vi "UI-抓边计算壁厚.vi"(8 "error in (no error)":errorcluster caption="错误输入（无错误）", 11 "名称或相对路径":string="Template Program") -> (0 "error in (no error) 2":errorcluster caption="错误输入（无错误）")   [LabVIEW 2017]
uses:
  Global System.vi
  <vilib>/Utility/xml.llb/Read From XML File(string).vi
  <vilib>/Utility/xml.llb/Write to XML File(string).vi
  Picture/SaveButtom.ctl
  <vilib>/vision/Measure.llb/Edge Polarity.ctl
  <vilib>/vision/Measure.llb/Edge Options.ctl
panel:
  out "添加的路径":path
  in  "刷新":bool
  in  "测试按钮":bool
  in  "保存按钮":bool
  in  "Main":enum32{"主参数", "计算圆心参数 ", "边界检查器设定", "测试效果"}(tab)
  in  "ParamsUI":T1={"IsNorImage"=TRUE, "Exposure Values"=100289, "ImagePath"=path "C:/Users/hedongpo/Desktop/514-hdp/Alignment Assemble System/Test Picture/B/3.bmp"} caption="参数界面" {"Exposure Values" scale=0.0..200000.0}
  in  "ParamsUI 内圆":T5={"圆参数1"={"Search  Direction"=0, "Edge Options"={"Edge Polarity"=0, "Kernel Size"=3, "Width"=3, "Minimum Edge Strength"=50.0, "Interpolation Type"=enum."Bilinear Fixed", "Data Processing Method"=enum."Average"}, "Show Search Area"=TRUE, "Show Search Lines"=TRUE, "Show Edges Found"=TRUE, "Show Result"=TRUE, "Search Area Color"=65280, "Search Lines Color"=255, "Edge Locations Color"=16776960, "Result Color"=16711680, "Overlay Group Name"=""}, "圆参数"={"Process"=enum."Get First Edge", "Step Size"=1, "Max Pixel Radius"=3}, "圆二值化设定"={"Lower value"=96.0, "Upper value"=255.0}, "圆环ROI设定"={"Center X"=1717, "Center Y"=1486, "Inner Radius"=327, "Outer Radius"=1645, "Start Angle"=0.0, "End Angle"=0.0}, "Show Search Area"=TRUE, "Show Search Lines"=TRUE, "Show Edges Found"=TRUE, "Show Result"=TRUE} caption="参数界面" {"圆环ROI设定"."End Angle" min=-90.0 max=90.0 step=1.0 format="%.2f"; "圆环ROI设定"."Start Angle" min=-90.0 max=90.0 step=1.0 format="%.2f"; "圆环ROI设定"."Center X" scale=0.0..1024.0; "圆参数1"."Search  Direction" items=["Outside to Inside", "Inside to Outside"]; "圆参数1"."Edge Options"."Edge Polarity" items=["All Edges", "Rising Edges", "Falling Edges"]; "圆参数1"."Edge Options"."Minimum Edge Strength" format="%.2f"; "圆参数1"."Edge Options"."Width" step=2; "圆参数1"."Edge Options"."Kernel Size" step=2}
  in  "ParamsUI 边界检查器":T6={"外圆二值化设定"={"Lower value"=96.0, "Upper value"=255.0}, "扇区个数"="1", "Process "=enum."Get All Edges", "Edge Options "={"Edge Polarity"=0, "Kernel Size"=9, "Width"=5, "Minimum Edge Strength"=27.0, "Interpolation Type"=enum."Bilinear", "Data Processing Method"=enum."Average"}} caption="参数界面" {"Edge Options"."Edge Polarity" items=["All Edges", "Rising Edges", "Falling Edges"]}
  out "壁厚波形图":sgl[](graph)
  in  "测试结果":string[][](table)=[["", ""]]
  out "原始图像":T7(plugin-control)
  out "处理后图像":T7(plugin-control)
  out "路径输出":path
  in  "Vision Paramter Save Buttom":T8
  out "system time":string
  in  "取消按钮":bool
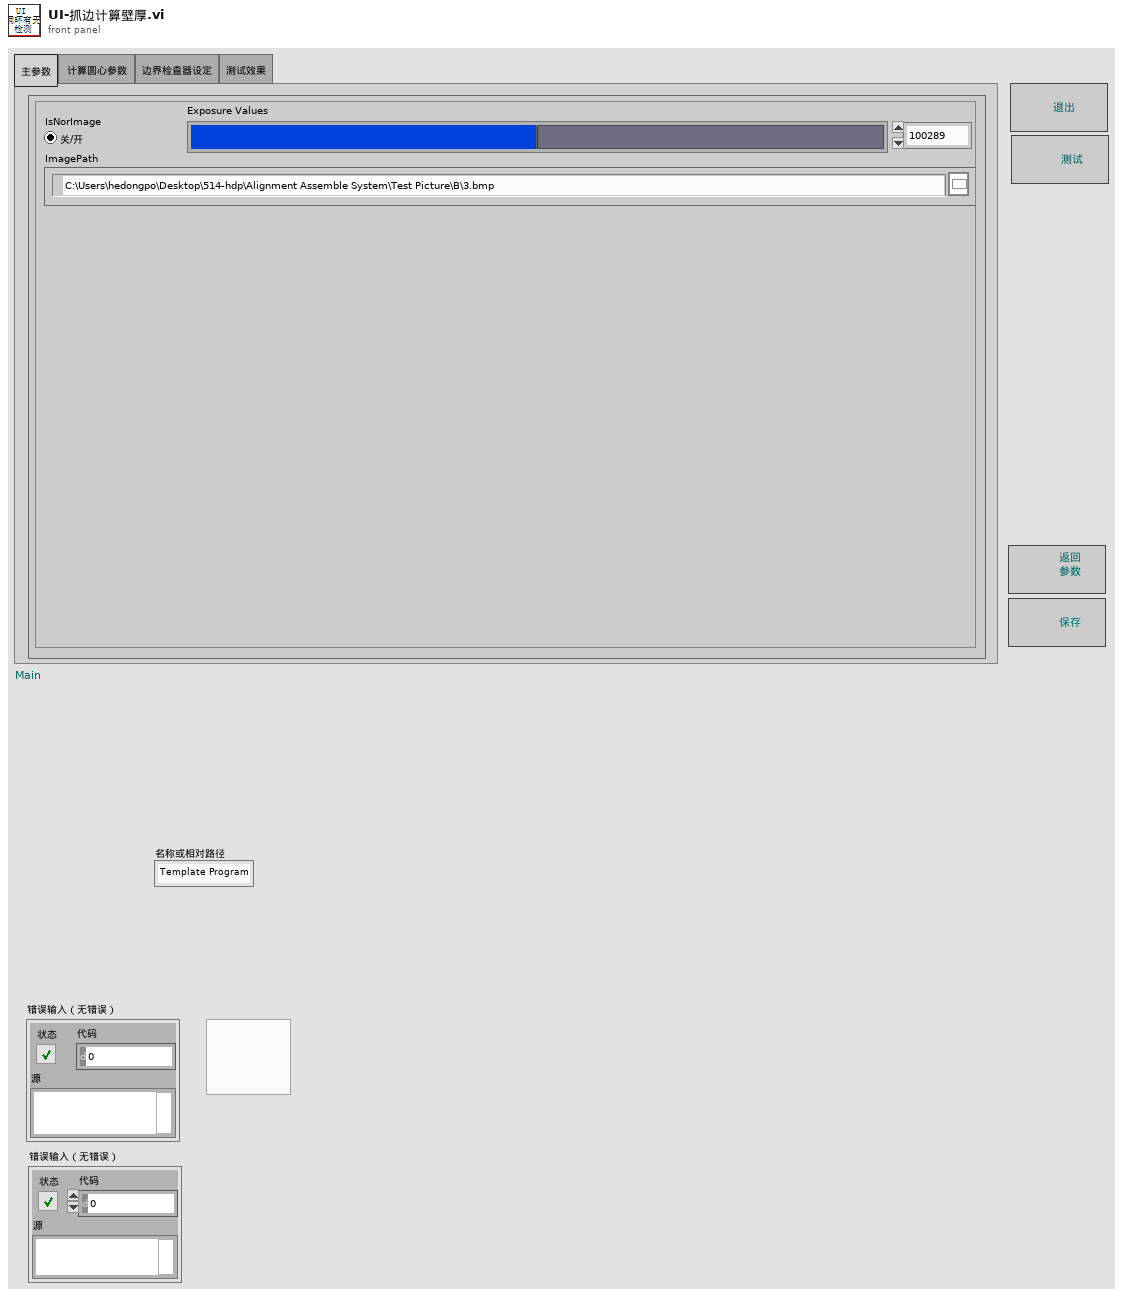
[diagram p1: front panel]
types:
  T1 = cluster{"IsNorImage":bool, "Exposure Values":u32, "ImagePath":path}
  T2 = typedef "Edge Options.ctl" = cluster{"Edge Polarity":T3, "Kernel Size":u32, "Width":u32, "Minimum Edge Strength":sgl, "Interpolation Type":enum32{"Zero Order", "Bilinear", "Quadratic", "Cubic", "Bilinear Fixed"}, "Data Processing Method":enum32{"Average", "Median"}}
  T3 = typedef "Edge Polarity.ctl" = u32
  T4 = typedef "IMAQ Circle" = cluster{"Center X":i32, "Center Y":i32, "Inner Radius":i32, "Outer Radius":i32, "Start Angle":dbl, "End Angle":dbl}
  T5 = cluster{"圆参数1":cluster{"Search  Direction":u32, "Edge Options":T2, "Show Search Area":bool, "Show Search Lines":bool, "Show Edges Found":bool, "Show Result":bool, "Search Area Color":u32, "Search Lines Color":u32, "Edge Locations Color":u32, "Result Color":u32, "Overlay Group Name":string}, "圆参数":cluster{"Process":enum16{"Get First Edge", "Get First + Last Edge", "Get All Edges", "Get Best Edge"}, "Step Size":i32, "Max Pixel Radius":i32}, "圆二值化设定":cluster{"Lower value":sgl, "Upper value":sgl}, "圆环ROI设定":T4, "Show Search Area":bool, "Show Search Lines":bool, "Show Edges Found":bool, "Show Result":bool}
  T6 = cluster{"外圆二值化设定":cluster{"Lower value":sgl, "Upper value":sgl}, "扇区个数":string, "Process ":enum16{"Get First Edge", "Get First + Last Edge", "Get All Edges", "Get Best Edge"}, "Edge Options ":cluster{"Edge Polarity":u32, "Kernel Size":u32, "Width":u32, "Minimum Edge Strength":sgl, "Interpolation Type":enum32{"Zero Order", "Bilinear", "Quadratic", "Cubic", "Bilinear Fixed"}, "Data Processing Method":enum32{"Average", "Median"}}}
  T7 = typedef "IMAQ Image.ctl" = refnum<image>
  T8 = typedef "SaveButtom.ctl" = bool
  T9 = cluster{"index":i32, "this vi":refnum<vi>, "error out":errorcluster}
  T10 = cluster{"master data":string, "priority":u16, "secondary data":string[]}
  T11 = cluster{"case name":string[], "queue array":refnum<queue>[]}
  T12 = cluster{"扇区个数":string, "Fitted Circle (Find Circular Edge 1)":cluster{"Center (Pixels)":cluster{"X":sgl, "Y":sgl}, "Radius (Pixels)":dbl, "Center (Real-World)":cluster{"X":sgl, "Y":sgl}, "Radius (Real-World)":dbl, "Roundness (Real-World)":dbl, "Average Strength":dbl, "Average SNR (dB)":dbl}, "Range (Threshold 1)":cluster{"Lower value":sgl, "Upper value":sgl}, "Process (Edge Detector 1)":enum16{"Get First Edge", "Get First + Last Edge", "Get All Edges", "Get Best Edge"}, "Edge Options (Edge Detector 1)":cluster{"Edge Polarity":u32, "Kernel Size":u32, "Width":u32, "Minimum Edge Strength":sgl, "Interpolation Type":enum32{"Zero Order", "Bilinear", "Quadratic", "Cubic", "Bilinear Fixed"}, "Data Processing Method":enum32{"Average", "Median"}}}
  T13 = typedef "Image Type" = u32
  T14 = cluster{"Search  Direction":u32, "Edge Options":T2, "Show Search Area":bool, "Show Search Lines":bool, "Show Edges Found":bool, "Show Result":bool, "Search Area Color":u32, "Search Lines Color":u32, "Edge Locations Color":u32, "Result Color":u32, "Overlay Group Name":string}
  T15 = cluster{"Process":enum16{"Get First Edge", "Get First + Last Edge", "Get All Edges", "Get Best Edge"}, "Step Size":i32, "Max Pixel Radius":i32}
  T16 = enum16{"Get First Edge", "Get First + Last Edge", "Get All Edges", "Get Best Edge"}
  T17 = cluster{"Edge Polarity":u32, "Kernel Size":u32, "Width":u32, "Minimum Edge Strength":sgl, "Interpolation Type":enum32{"Zero Order", "Bilinear", "Quadratic", "Cubic", "Bilinear Fixed"}, "Data Processing Method":enum32{"Average", "Median"}}
  T18 = typedef "ROI Descriptor" = cluster{"Global Rectangle":i32[], "Contours":cluster{"ID":enum32{"External", "Internal"}, "Type":u32, "Coordinates":i32[]}[]}
  T19 = cluster{"Center (Pixels)":cluster{"X":sgl, "Y":sgl}, "Radius (Pixels)":dbl, "Center (Real-World)":cluster{"X":sgl, "Y":sgl}, "Radius (Real-World)":dbl, "Roundness (Real-World)":dbl, "Average Strength":dbl, "Average SNR (dB)":dbl}
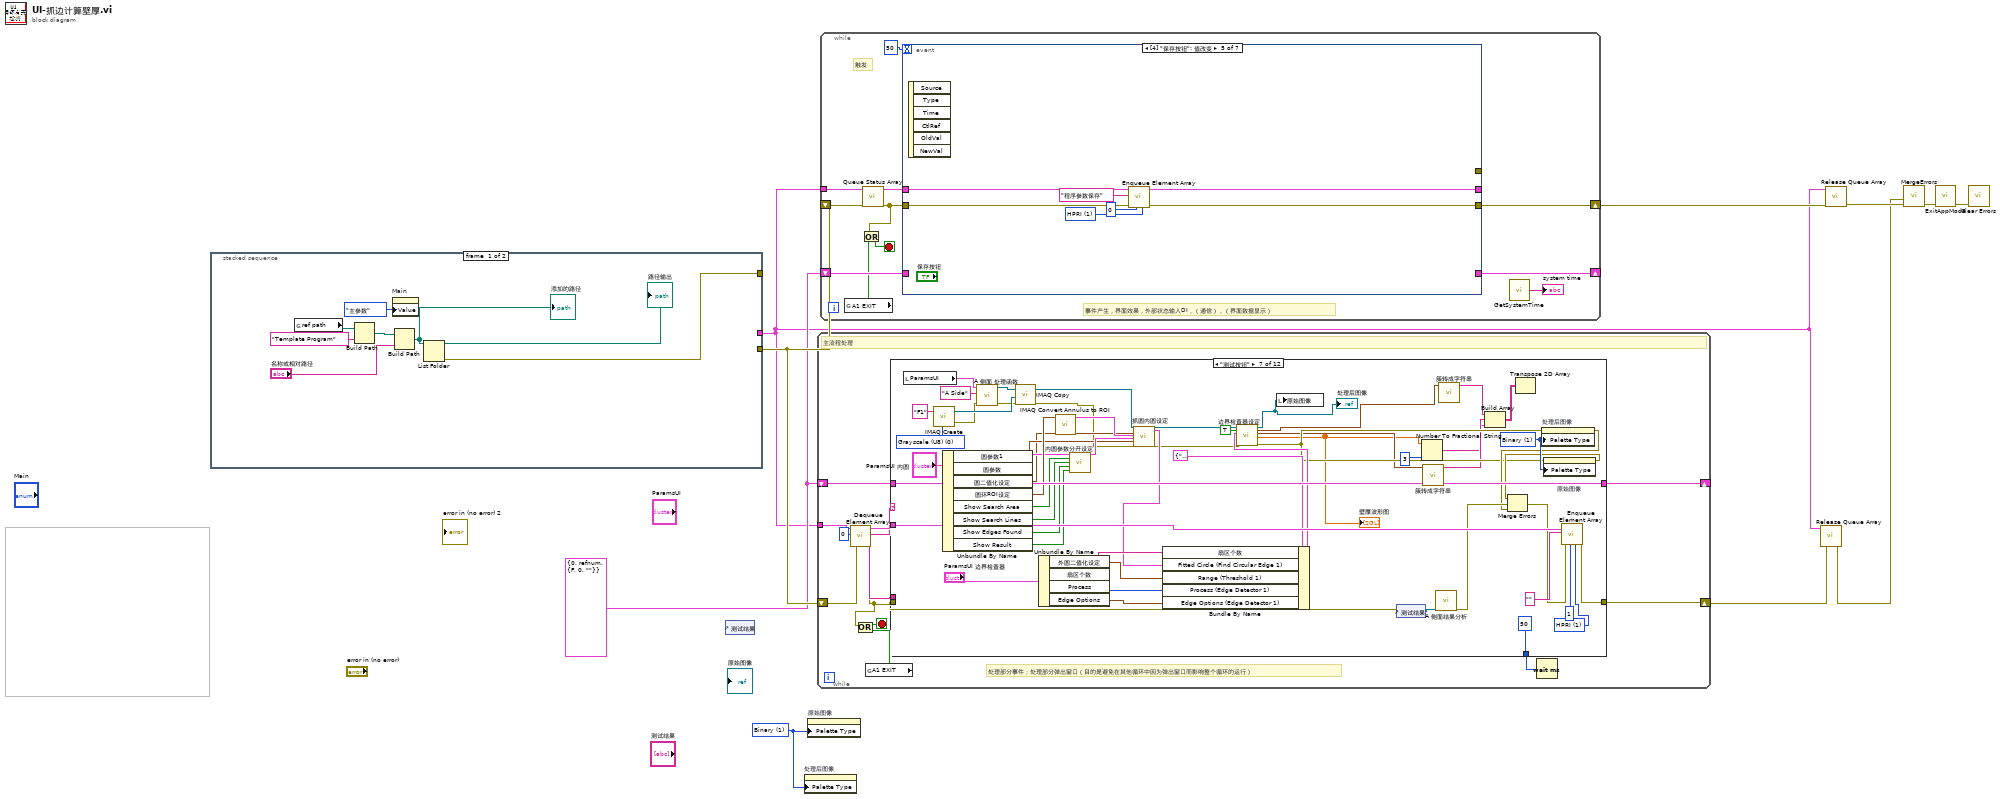
[diagram p0: block diagram]
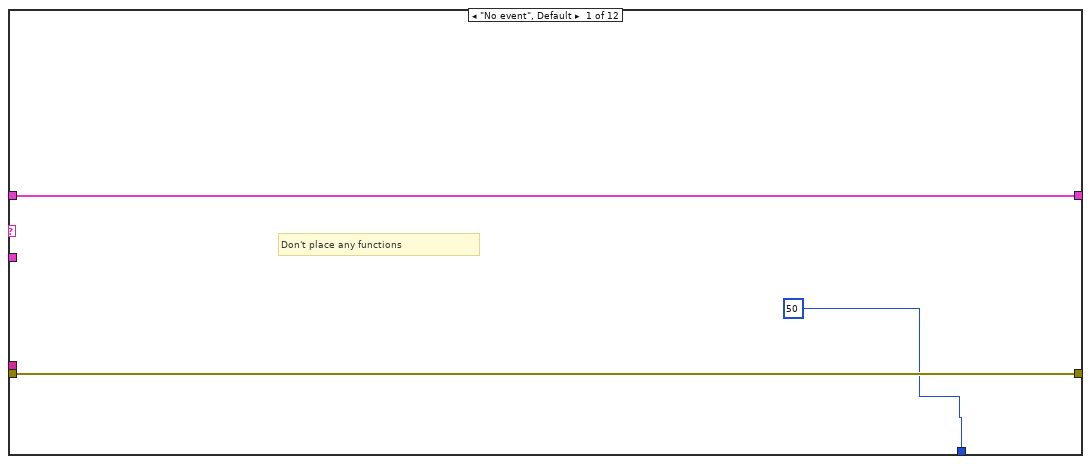
[diagram p2: hidden frame]
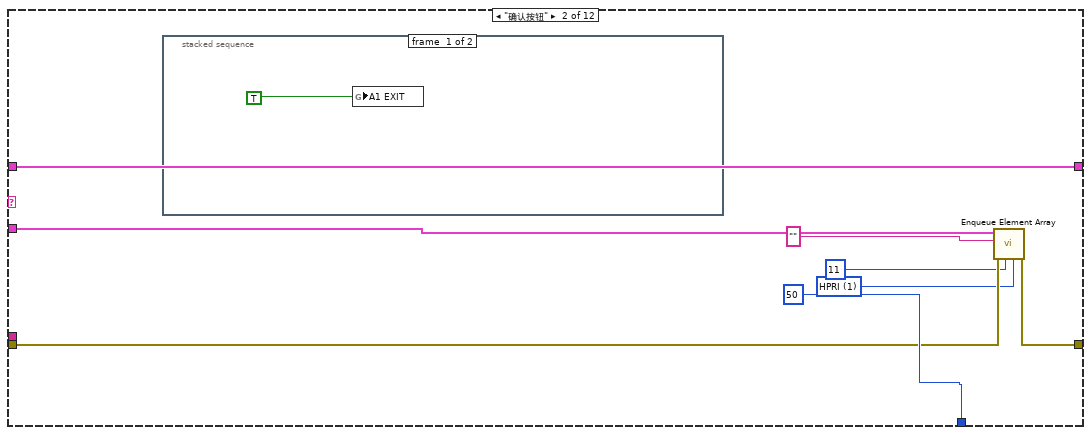
[diagram p3: hidden frame]
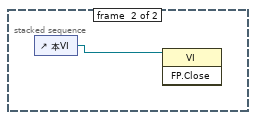
[diagram p4: hidden frame]
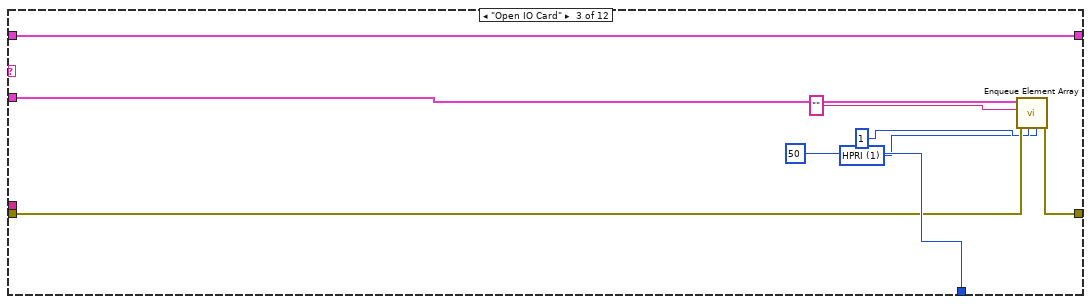
[diagram p5: hidden frame]
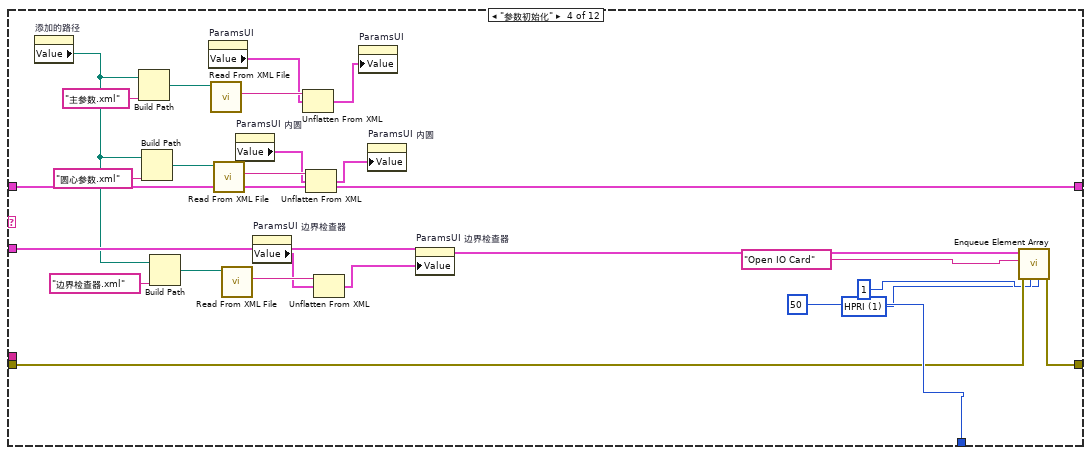
[diagram p6: hidden frame]
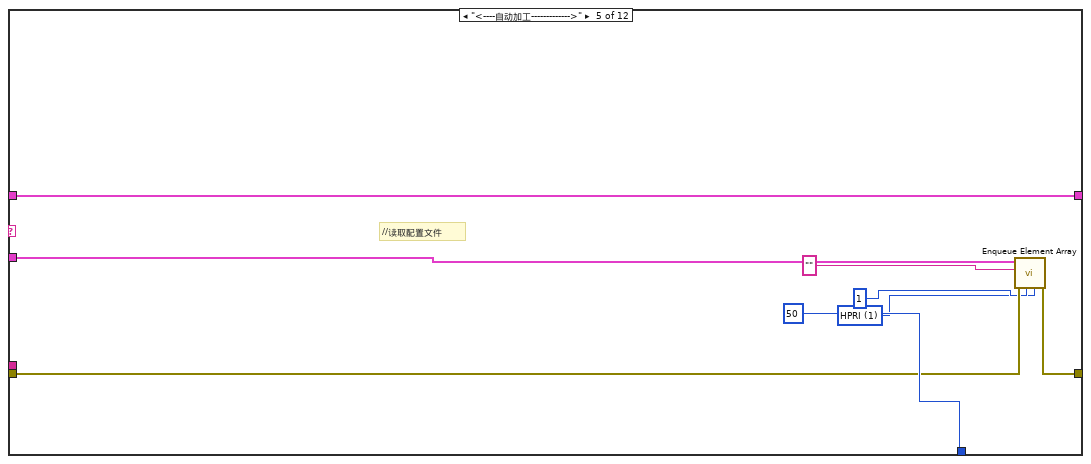
[diagram p7: hidden frame]
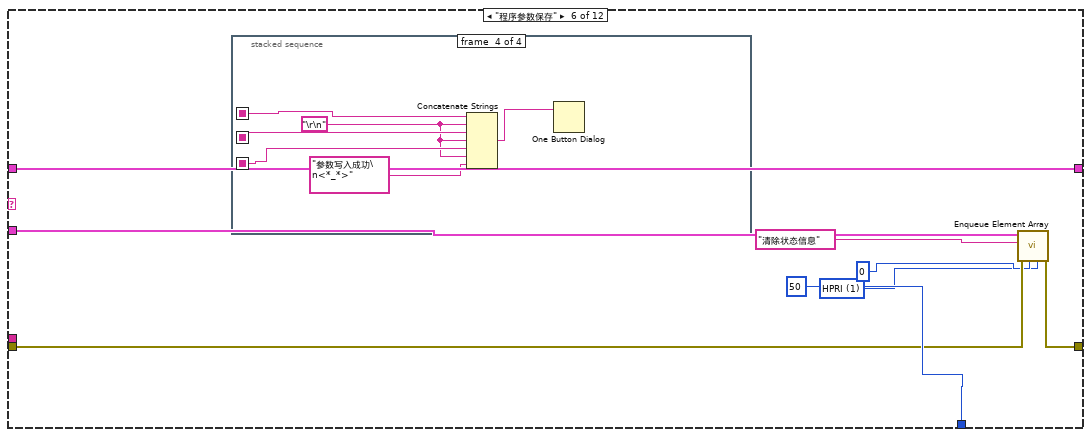
[diagram p8: hidden frame]
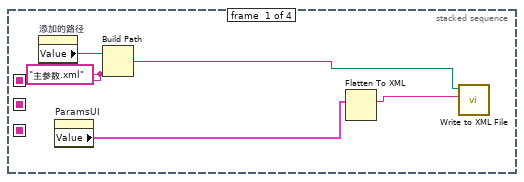
[diagram p9: hidden frame]
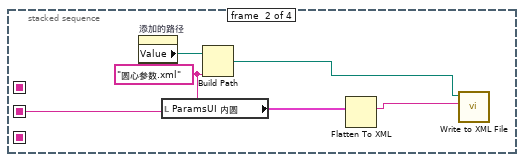
[diagram p10: hidden frame]
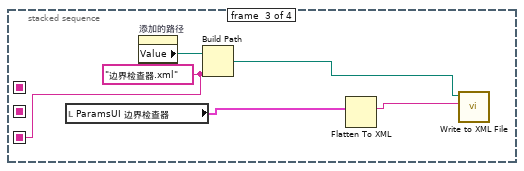
[diagram p11: hidden frame]
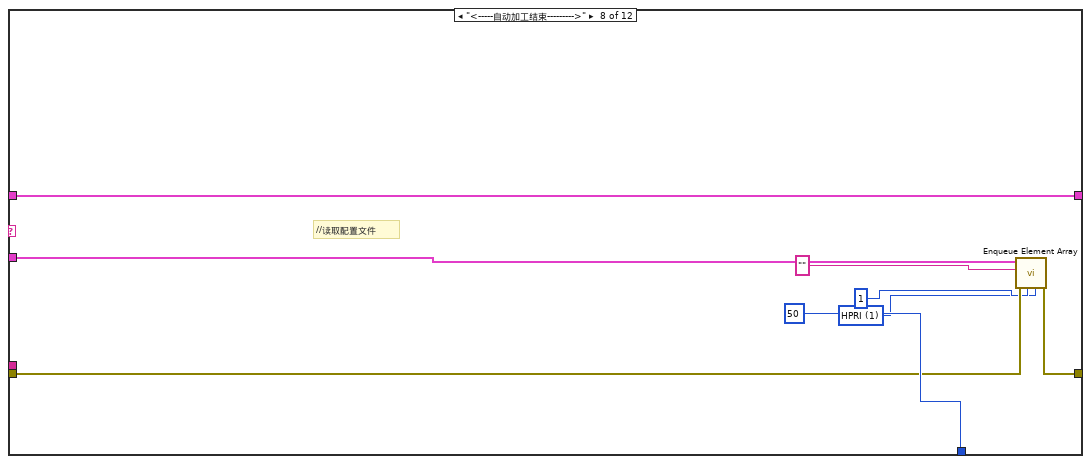
[diagram p12: hidden frame]
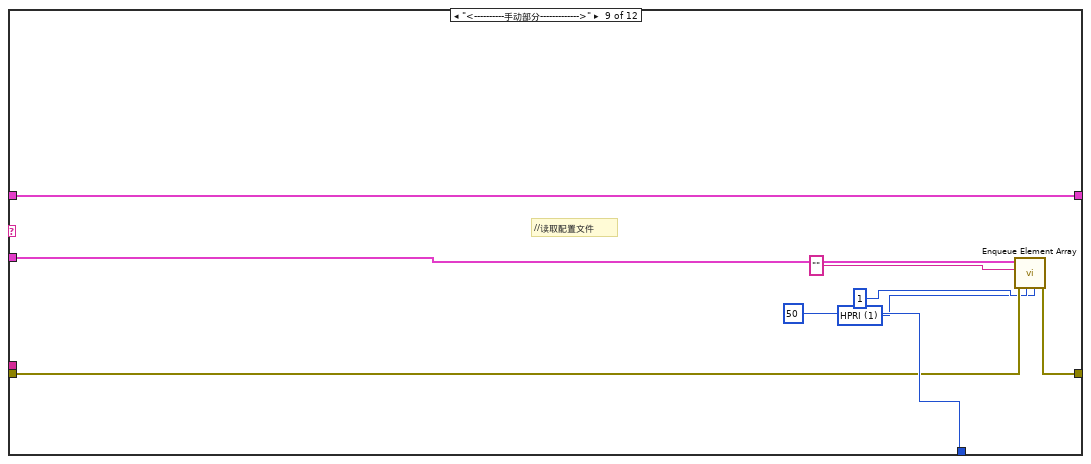
[diagram p13: hidden frame]
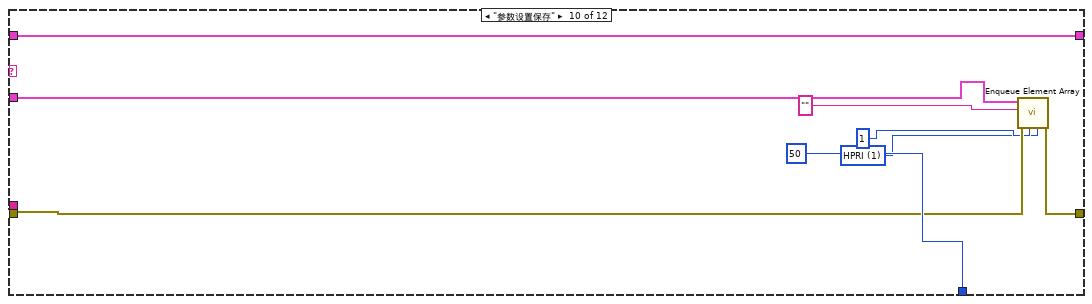
[diagram p14: hidden frame]
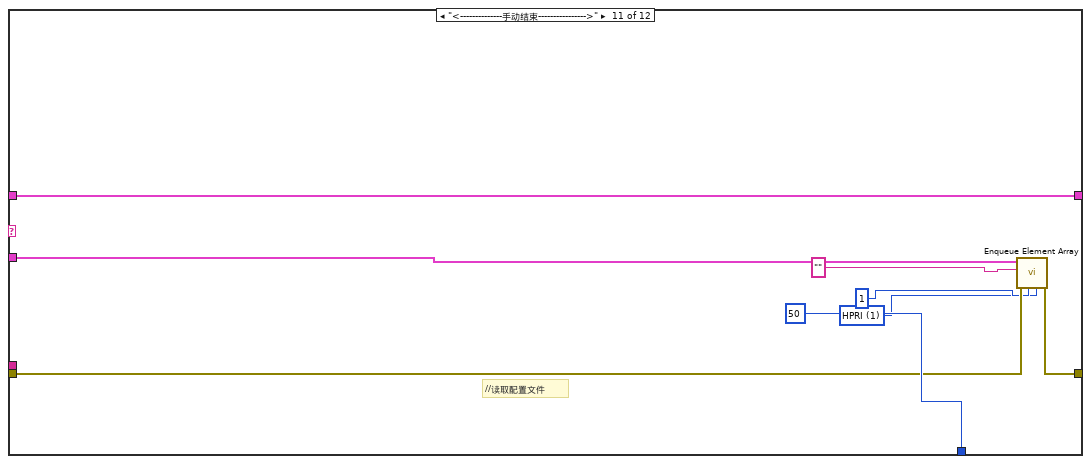
[diagram p15: hidden frame]
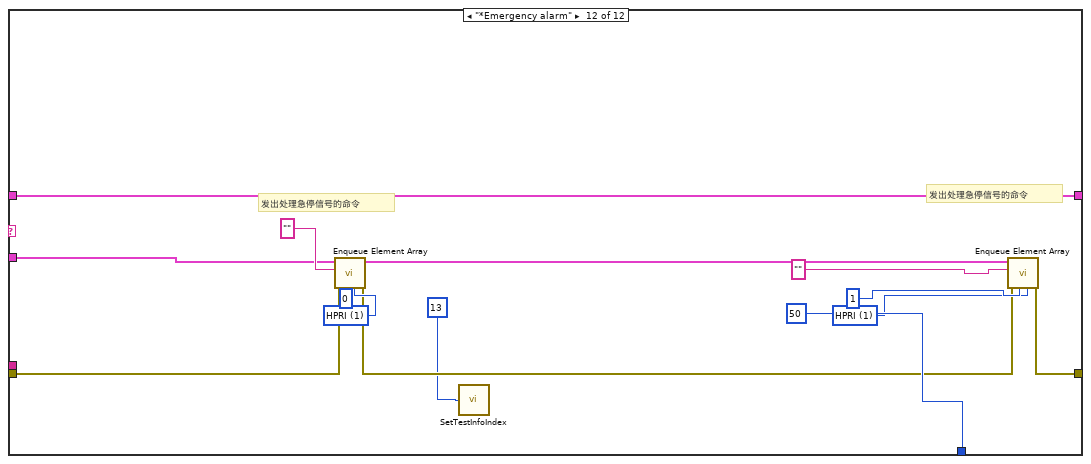
[diagram p16: hidden frame]
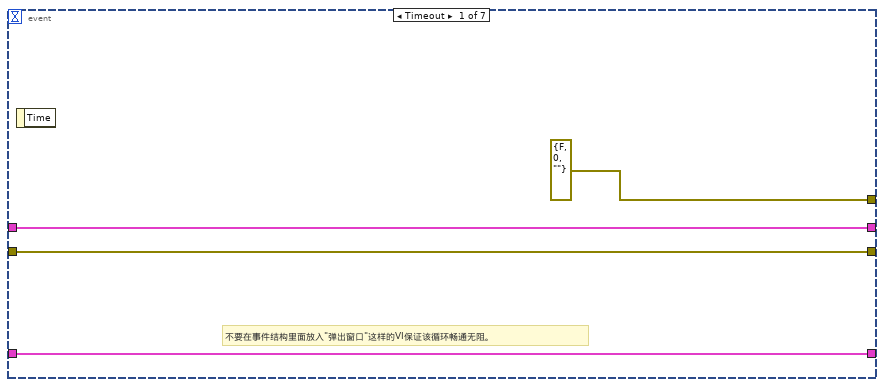
[diagram p17: hidden frame]
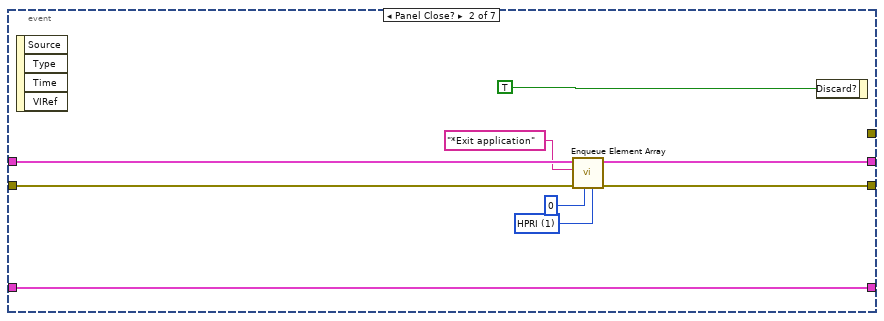
[diagram p18: hidden frame]
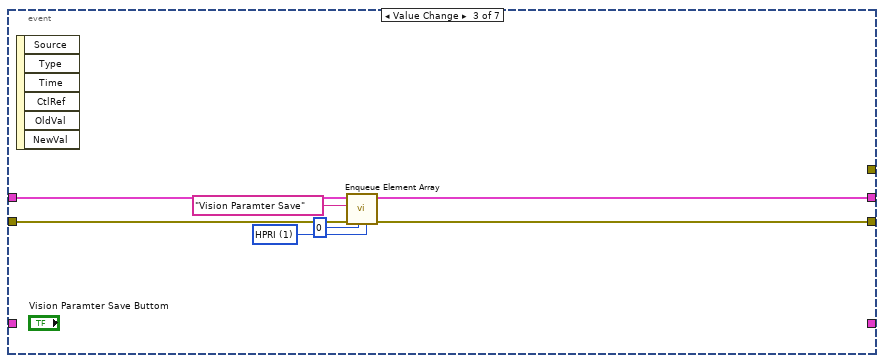
[diagram p19: hidden frame]
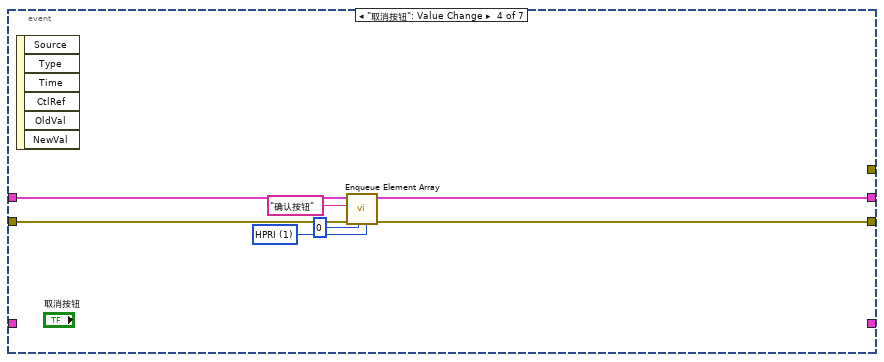
[diagram p20: hidden frame]
diagram:
  w1 = u32 1 items=["Grayscale", "Binary", "Gradient", "Rainbow", "Temperature", "User Defined", "Binary 16 Bit", "Gradient 16 Bit", "Rainbow 16 Bit", "Temperature 16 Bit", "User Defined 16 Bit"] ("Palette:Palette Type")
  w5 = T9 {"index"=0, "this vi"=refnum, "error out"={"status"=FALSE, "code"=0, "source"=""}} ("parameter buffer")
  n1 = stacked-sequence {
    tunnel: [w16 _] -> _
    tunnel: [_ w20] -> w6
    tunnel: [_ w19] -> w2
    frame #0 {
      n2 = global read "Global System.vi" "ref path"() -> (w14:path)
      n3 = Build Path(base path=w14, name or relative path="Template Program" ("名称或相对路径")) -> (appended path=w12:path)
      n4 = property on="Main" class="TabCtl (严格)"("Value"=enum32{"主参数", "计算圆心参数 ", "边界检查器设定", "测试效果"}."主参数" ("Main")) -> ()  [unwired: 2 in, 2 out]
      n5 = Build Path(base path=w12, name or relative path="名称或相对路径") -> (appended path=w18:path)
      "添加的路径" <- w18
      n6 = List Folder(path=w18) -> (path out=→"路径输出":path, error out=w16:errorcluster)  [unwired: 3 in, 2 out]
    }
    frame #1 {
      w28 = string[] ["comm queue1", "data queue 11", "data queue 12", "data queue 13", "data queue 14"]  # queue name
      w29 = 4  # queue num
      w30 = T10 {"master data"="", "priority"=0, "secondary data"=[]}  # element data type
      n7 = call "Obtain Queue Array.vi"("queue name"=w28, "element data type"=w30, "queue num"=w29) -> ("error out"=w24:errorcluster, "queue out"=w25:T11)  [unwired: 2 in, 1 out]
      n8 = call "Enqueue Element Array.vi"("queue index"=0, "error in"=w24, "master data"="参数初始化", "queue in"=w25) -> ("error out"=w23:errorcluster, "queue out"=w22:T11)  [unwired: 6 in]
      n9 = disable-structure shown="启用" {
        disable-tunnel: w23 -> [w36 w37]
        disable-tunnel: w22 -> [w35 w38]
        disable-tunnel: "Loading Variable" ("master data") -> [w34 _]
        disable-tunnel: [w32 w37] -> w20
        disable-tunnel: [w31 w38] -> w19
        frame Disabled {
          n10 = call "Enqueue Element Array.vi"("queue index"=12, "error in"=w36, "master data"=w34, "queue in"=w35) -> ("error out"=w32:errorcluster, "queue out"=w31:T11)  [unwired: 6 in]
        }
        frame Enabled {
        }
      }
    }
  }
  n11 = control-ref of="测试结果"() -> ()  [unwired: 1 out]
  n12 = property on="处理后图像" class="ImageControl"("Palette Type"=w1) -> ()  [unwired: 2 in, 2 out]
  n13 = property on="原始图像" class="ImageControl"("Palette Type"=w1) -> ()  [unwired: 2 in, 2 out]
  n14 = while {
    shift-right: [w51] -> w4
    shift-left: w6 -> [w42]
    shift-right: [w48] -> _
    shift-left: w5 -> [w49]
    tunnel: w2 -> [w44]
    stop <- w39 stop-if-true
    # "处理部分事件；处理部分弹出窗口（目的是避免在其他循环中因为弹出窗口而影响整个循环的运行）"
    # "主流程处理"
    n15 = call "Dequeue Element Array.vi"("queue in"=w44, "queue index"=0, "error in"=w42) -> ("queue out"=w47:T11, "master data"=w46:string, "secondary data"=w45:string[], "error out"=w41:errorcluster)  [unwired: 2 in, 1 out]
    n16 = global read "Global System.vi" "A1 EXIT"() -> (w40:bool)
    n17 = Or(x=w41, y=w40) -> (x .or. y?=w39:bool)
    n18 = case shown="\"测试按钮\"" w46 {
      tunnel: w47 -> [_ w61 w71 w95 w103 w105 w187 w195 w203 w211 w219 w225]
      tunnel: w41 -> [w53 w57 w67 w92 w99 w109 w170 w191 w199 w207 w215 w222]
      tunnel: [w53 w60 w70 w94 w102 w111 w186 w194 w202 w210 w218 w233] -> w51
      tunnel: [50 50 50 50 50 50 50 50 50 50 50 50] -> w50
      tunnel: w49 -> [w54 w58 w68 w89 w100 w106 w182 w192 w200 w208 w216 w231]
      tunnel: [w54 w58 w68 w89 w100 w106 w182 w192 w200 w208 w216 w231] -> w48
      tunnel: w45 -> [_ _ _ _ _ _ _ _ _ _ _ _]
      frame "No event", Default {
        # "Don't place any functions"
      }
      frame "确认按钮" {
        w55 = u16 1 items=["HPRI"=1, "LPRI"=0] ("priority")
        n19 = stacked-sequence {
          frame #0 {
            n20 = global write "Global System.vi" "A1 EXIT"(TRUE ("EXIT")) -> ()
          }
          frame #1 {
            n21 = control-ref of="本VI"() -> (w64:refnum<vi>)
            n22 = invoke class="VI" method="FP.Close"(reference=w64) -> ()  [unwired: 2 in, 3 out]
          }
        }
        n23 = call "Enqueue Element Array.vi"("priority"=w55, "queue index"=11, "error in"=w57, "master data"="" ("Element 1"), "queue in"=w61) -> ("error out"=w60:errorcluster)  [unwired: 5 in, 1 out]
      }
      frame "Open IO Card" {
        w65 = u16 1 items=["HPRI"=1, "LPRI"=0] ("priority")
        n24 = call "Enqueue Element Array.vi"("priority"=w65, "queue index"=1, "error in"=w67, "master data"="" ("Element 1"), "queue in"=w71) -> ("error out"=w70:errorcluster)  [unwired: 5 in, 1 out]
      }
      frame "参数初始化" {
        w90 = u16 1 items=["HPRI"=1, "LPRI"=0] ("priority")
        n25 = property on="添加的路径" class="Path"() -> ("Value"=w75:path)  [unwired: 2 in, 2 out]
        n26 = Build Path(base path=w75, name or relative path="主参数.xml" ("名称或相对路径")) -> (appended path=w87:path)
        n27 = Build Path(base path=w75, name or relative path="圆心参数.xml" ("名称或相对路径")) -> (appended path=w82:path)
        n28 = Build Path(base path=w75, name or relative path="边界检查器.xml" ("名称或相对路径")) -> (appended path=w77:path)
        n29 = property on="ParamsUI" class="Clust (严格)"() -> ("Value"=w85:T1)  [unwired: 2 in, 2 out]
        n30 = call-poly <vilib>:"Read From XML File.vi"("XML File Path"=w87) -> ("XML Elements"=w86:string)  [unwired: 8 in, 2 out]
        n31 = call-poly <vilib>:"Read From XML File.vi"("XML File Path"=w82) -> ("XML Elements"=w83:string)  [unwired: 8 in, 2 out]
        n32 = call-poly <vilib>:"Read From XML File.vi"("XML File Path"=w77) -> ("XML Elements"=w76:string)  [unwired: 8 in, 2 out]
        n33 = property on="ParamsUI 内圆" class="Clust (严格)"() -> ("Value"=w80:T5)  [unwired: 2 in, 2 out]
        n34 = property on="ParamsUI 边界检查器" class="Clust (严格)"() -> ("Value"=w74:T6)  [unwired: 2 in, 2 out]
        n35 = Unflatten From XML(xml string=w86, type=w85) -> (value=w84:T1)  [unwired: 1 in, 1 out]
        n36 = Unflatten From XML(xml string=w83, type=w80) -> (value=w79:T5)  [unwired: 1 in, 1 out]
        n37 = Unflatten From XML(xml string=w76, type=w74) -> (value=w73:T6)  [unwired: 1 in, 1 out]
        n38 = property on="ParamsUI" class="Clust (严格)"("Value"=w84) -> ()  [unwired: 2 in, 2 out]
        n39 = property on="ParamsUI 内圆" class="Clust (严格)"("Value"=w79) -> ()  [unwired: 2 in, 2 out]
        n40 = property on="ParamsUI 边界检查器" class="Clust (严格)"("Value"=w73) -> ()  [unwired: 2 in, 2 out]
        n41 = call "Enqueue Element Array.vi"("priority"=w90, "queue index"=1, "error in"=w92, "master data"="Open IO Card" ("Element 1"), "queue in"=w95) -> ("error out"=w94:errorcluster)  [unwired: 5 in, 1 out]
      }
      frame "<----自动加工------------->" {
        w97 = u16 1 items=["HPRI"=1, "LPRI"=0] ("priority")
        # "//读取配置文件"
        n42 = call "Enqueue Element Array.vi"("priority"=w97, "queue index"=1, "error in"=w99, "master data"="" ("Element 1"), "queue in"=w103) -> ("error out"=w102:errorcluster)  [unwired: 5 in, 1 out]
      }
      frame "程序参数保存" {
        w107 = u16 1 items=["HPRI"=1, "LPRI"=0] ("priority")
        n43 = stacked-sequence {
          seq-local: [w113 _ _ _] -> [_ _ _ w132]
          seq-local: [_ w118 _ _] -> [_ _ _ w130]
          seq-local: [_ _ w124 _] -> [_ _ _ w129]
          frame #0 {
            w113 = "主参数.xml" ("名称或相对路径")
            n44 = property on="添加的路径" class="Path"() -> ("Value"=w117:path)  [unwired: 2 in, 2 out]
            n45 = property on="ParamsUI" class="Clust (严格)"() -> ("Value"=w116:T1)  [unwired: 2 in, 2 out]
            n46 = Build Path(base path=w117, name or relative path=w113) -> (appended path=w114:path)
            n47 = Flatten To XML(anything=w116) -> (xml string=w115:string)
            n48 = call-poly <vilib>:"Write to XML File.vi"("XML Input"=w115, "XML File Path"=w114) -> ()  [unwired: 7 in, 3 out]
          }
          frame #1 {
            w118 = "圆心参数.xml" ("名称或相对路径")
            n49 = property on="添加的路径" class="Path"() -> ("Value"=w122:path)  [unwired: 2 in, 2 out]
            n50 = local read "ParamsUI 内圆"() -> (w119:T5)
            n51 = Build Path(base path=w122, name or relative path=w118) -> (appended path=w120:path)
            n52 = Flatten To XML(anything=w119) -> (xml string=w121:string)
            n53 = call-poly <vilib>:"Write to XML File.vi"("XML Input"=w121, "XML File Path"=w120) -> ()  [unwired: 7 in, 3 out]
          }
          frame #2 {
            w124 = "边界检查器.xml" ("名称或相对路径")
            n54 = local read "ParamsUI 边界检查器"() -> (w123:T6)
            n55 = property on="添加的路径" class="Path"() -> ("Value"=w127:path)  [unwired: 2 in, 2 out]
            n56 = Build Path(base path=w127, name or relative path=w124) -> (appended path=w125:path)
            n57 = Flatten To XML(anything=w123) -> (xml string=w126:string)
            n58 = call-poly <vilib>:"Write to XML File.vi"("XML Input"=w126, "XML File Path"=w125) -> ()  [unwired: 7 in, 3 out]
          }
          frame #3 {
            w128 = "\r\n"
            n59 = Concatenate Strings(w132, w128, w130, w128, w129, w128, "参数写入成功\n<*_*>" ("消息")) -> (w131:string)
            n60 = One Button Dialog(message=w131) -> ()  [unwired: 1 in, 1 out]
          }
        }
        n61 = call "Enqueue Element Array.vi"("priority"=w107, "queue index"=0, "error in"=w109, "master data"="清除状态信息" ("Element 1"), "queue in"=w105) -> ("error out"=w111:errorcluster)  [unwired: 5 in, 1 out]
      }
      frame "测试按钮" {
        w173 = u32 1 items=["Grayscale", "Binary", "Gradient", "Rainbow", "Temperature", "User Defined", "Binary 16 Bit", "Gradient 16 Bit", "Rainbow 16 Bit", "Temperature 16 Bit", "User Defined 16 Bit"] ("Palette:Palette Type")
        w180 = T13 0 items=["Grayscale (U8)", "Grayscale (I16)", "Grayscale (SGL)", "Complex (CSG)", "RGB (U32)", "HSL (U32)", "RGB (U64)", "Grayscale (U16)"] ("Image Type")
        w183 = u16 1 items=["HPRI"=1, "LPRI"=0] ("priority")
        n62 = local read "ParamsUI"() -> (w172:T1)
        n63 = call "IMAQ Create"("Image Name"="F1", "Image Type"=w180) -> ("New Image"=w179:T7, "error out"=w177:errorcluster)  [unwired: 3 in]
        n64 = Unbundle By Name("ParamsUI 内圆") -> ("圆参数1"=w162:T14, "圆参数"=w160:T15, "圆二值化设定"=w159:cluster{"Lower value":sgl, "Upper value":sgl}, "圆环ROI设定"=w163:T4, "Show Search Area"=w158:bool, "Show Search Lines"=w157:bool, "Show Edges Found"=w156:bool, "Show Result"=w155:bool)
        n65 = call "A 侧面 处理函数.vi"("error in (no error)"=w177, "Image Name"="A Side", "ParamsUI"=w172) -> ("error out"=w175:errorcluster, "Image out"=w176:T7)  [unwired: 5 in, 2 out]
        n66 = call "IMAQ Copy"("error in (no error)"=w175, "Image Dst"=w179, "Image Src"=w176) -> ("error out"=w144:errorcluster, "Image Dst Out"=w161:T7)  [unwired: 3 in]
        n67 = Unbundle By Name("ParamsUI 边界检查器") -> ("外圆二值化设定"=w135:cluster{"Lower value":sgl, "Upper value":sgl}, "扇区个数"=w149:string, "Process"=w148:T16, "Edge Options"=w147:T17)
        n68 = call "IMAQ Convert Annulus to ROI"("Annulus"=w163) -> ("ROI Descriptor"=w164:T18)  [unwired: 8 in, 1 out]
        n69 = call "内圆参数分开设定.vi"("内圆参数in"=w162, "Show Search Area"=w158, "Show Search Lines"=w157, "Show Edges Found"=w156, "Show Result"=w155) -> ("our"=w166:T14)  [unwired: 10 in]
        n70 = call "抓圆内圆设定"("Image In"=w161, "Range (Threshold 1)"=w159, "ROI Descriptor (Find Circular Edge 1)"=w164, "Options (Find Circular Edge 1)"=w166, "Circle Fit Options (Find Circular Edge 1)"=w160, "error in"=w144) -> ("Image Out"=w154:T7, "Fitted Circle (Find Circular Edge 1)"=w146:T19, "error out"=w143:errorcluster)  [unwired: 19 in]
        n71 = Bundle By Name(cluster=T12 {"扇区个数"="1", "Fitted Circle (Find Circular Edge 1)"={"Center (Pixels)"={"X"=1736.0, "Y"=1501.0}, "Radius (Pixels)"=1442.0, "Center (Real-World)"={"X"=1736.0, "Y"=1501.0}, "Radius (Real-World)"=1442.0, "Roundness (Real-World)"=0.0, "Average Strength"=0.0, "Average SNR (dB)"=0.0}, "Range (Threshold 1)"={"Lower value"=65.0, "Upper value"=255.0}, "Process (Edge Detector 1)"=enum."Get All Edges", "Edge Options (Edge Detector 1)"={"Edge Polarity"=0, "Kernel Size"=9, "Width"=5, "Minimum Edge Strength"=27.0, "Interpolation Type"=enum."Bilinear", "Data Processing Method"=enum."Average"}} ("边界检查器参数"), "扇区个数"=w149, "Fitted Circle (Find Circular Edge 1)"=w146, "Range (Threshold 1)"=w135, "Process (Edge Detector 1)"=w148, "Edge Options (Edge Detector 1)"=w147) -> (w145:T12)
        n72 = call "边界检查器设定.vi"("Image IN"=w154, "启动变量"=TRUE, "边界检查器参数"=w145, "error in"=w143) -> ("Image Out"=w153:T7, "起始点"=w141:cluster{"X":sgl, "Y":sgl}[], "结束点"=w139:cluster{"X":sgl, "Y":sgl}[], "厚度"=w134:sgl[], "error out"=w142:errorcluster)  [unwired: 11 in]
        "处理后图像" <- w153
        "壁厚波形图" <- w134
        n73 = local write "原始图像"(w153) -> ()
        n74 = control-ref of="测试结果"() -> (w174:refnum<vi>)
        n75 = Number To Fractional String(number=w134, precision (6)=i16 3 ("精度(6)")) -> (F-format string=w137:string[])  [unwired: 2 in]
        n76 = call "簇转成字符串.vi"("起始点"=w139) -> ("字符串"=w138:string[])  [unwired: 10 in]
        n77 = call "A 侧面结果分析.vi"("Tbl引用句柄"=w174) -> ()  [unwired: 11 in]
        n78 = call "簇转成字符串.vi"("起始点"=w141) -> ("字符串"=w140:string[])  [unwired: 10 in]
        n79 = Build Array(w140, w138, w137) -> (w136:string[][])
        n80 = Transpose 2D Array(2D array=w136) -> ()  [unwired: 1 out]
        n81 = property on="处理后图像" class="ImageControl"(error in=w142, "Palette Type"=w173) -> (error out=w168:errorcluster)  [unwired: 1 in, 1 out]
        n82 = property on="原始图像" class="ImageControl"(error in=w142, "Palette Type"=w173) -> (error out=w171:errorcluster)  [unwired: 1 in, 1 out]
        n83 = Merge Errors(w171, w170, w168) -> (w169:errorcluster)
        n84 = call "Enqueue Element Array.vi"("priority"=w183, "queue index"=1, "error in"=w169, "master data"="" ("Element 1"), "queue in"=w187) -> ("error out"=w186:errorcluster)  [unwired: 5 in, 1 out]
      }
      frame "<-----自动加工结束--------->" {
        w189 = u16 1 items=["HPRI"=1, "LPRI"=0] ("priority")
        # "//读取配置文件"
        n85 = call "Enqueue Element Array.vi"("priority"=w189, "queue index"=1, "error in"=w191, "master data"="" ("Element 1"), "queue in"=w195) -> ("error out"=w194:errorcluster)  [unwired: 5 in, 1 out]
      }
      frame "<----------手动部分------------->" {
        w197 = u16 1 items=["HPRI"=1, "LPRI"=0] ("priority")
        # "//读取配置文件"
        n86 = call "Enqueue Element Array.vi"("priority"=w197, "queue index"=1, "error in"=w199, "master data"="" ("Element 1"), "queue in"=w203) -> ("error out"=w202:errorcluster)  [unwired: 5 in, 1 out]
      }
      frame "参数设置保存" {
        w205 = u16 1 items=["HPRI"=1, "LPRI"=0] ("priority")
        n87 = call "Enqueue Element Array.vi"("priority"=w205, "queue index"=1, "error in"=w207, "master data"="" ("Element 1"), "queue in"=w211) -> ("error out"=w210:errorcluster)  [unwired: 5 in, 1 out]
      }
      frame "<--------------手动结束---------------->" {
        w213 = u16 1 items=["HPRI"=1, "LPRI"=0] ("priority")
        # "//读取配置文件"
        n88 = call "Enqueue Element Array.vi"("priority"=w213, "queue index"=1, "error in"=w215, "master data"="" ("Element 1"), "queue in"=w219) -> ("error out"=w218:errorcluster)  [unwired: 5 in, 1 out]
      }
      frame "*Emergency alarm" {
        w228 = u16 1 items=["HPRI"=1, "LPRI"=0] ("priority")
        w229 = u16 1 items=["HPRI"=1, "LPRI"=0] ("priority")
        # "发出处理急停信号的命令"
        # "发出处理急停信号的命令"
        n89 = call "Enqueue Element Array.vi"("priority"=w228, "queue index"=0, "error in"=w222, "master data"="" ("Element 1"), "queue in"=w225) -> ("error out"=w223:errorcluster, "queue out"=w224:T11)  [unwired: 5 in]
        n90 = call "SetTestInfoIndex.vi"("test info index"=13) -> ()
        n91 = call "Enqueue Element Array.vi"("priority"=w229, "queue index"=1, "error in"=w223, "master data"="" ("Element 1"), "queue in"=w224) -> ("error out"=w233:errorcluster)  [unwired: 5 in, 1 out]
      }
    }
    n92 = Wait (ms)(milliseconds to wait=w50) -> ()  [unwired: 1 out]
  }
  n93 = while {
    shift-right: [w238] -> w7
    shift-left: w6 -> [w242]
    shift-right: [w240] -> _
    shift-left: w5 -> [w241]
    tunnel: w2 -> [w244]
    stop <- w235 stop-if-true
    # "触发"
    # "事件产生，界面效果，外部状态输入DI，（通信），（界面数据显示）"
    n94 = global read "Global System.vi" "A1 EXIT"() -> (w236:bool)
    n95 = call "Queue Status Array.vi"("error in (no error)"=w242, "queue in"=w244) -> ("error out"=w237:errorcluster, "queue out"=w239:T11)  [unwired: 4 in]
    n96 = Or(x=w237, y=w236) -> (x .or. y?=w235:bool)
    n97 = event shown="[4] \"保存按钮\": 值改变" {
      selector: _ -> [_ _ _ _ _ _ _]
      dyn-events: _ -> [_ _ _ _ _ _ _]
      timeout: 50 -> [_ _ _ _ _ _ _]
      tunnel: w241 -> [w249 w257 _ _ _ _ _]
      tunnel: [w249 w257 _ _ _ _ _] -> w240
      tunnel: [errorcluster {"status"=FALSE, "code"=0, "source"=""} ("error out") _ _ _ _ _ _] -> _
      tunnel: w239 -> [w247 w256 w262 w269 w276 w284 w292]
      tunnel: w237 -> [w246 w255 w261 w268 w275 w283 w291]
      tunnel: [w246 w254 w259 w266 w273 w281 w289] -> w238
      tunnel: [w247 w253 w260 w267 w274 w282 w290] -> _
      event Timeout {
        # "不要在事件结构里面放入\"弹出窗口\"这样的VI保证该循环畅通无阻。"
        n98 = event-data() -> ()  [unwired: 1 in, 1 out]
      }
      event Panel Close? {
        w251 = u16 1 items=["HPRI"=1, "LPRI"=0] ("priority")
        n99 = event-data() -> ()  [unwired: 1 in, 4 out]
        n100 = call "Enqueue Element Array.vi"("priority"=w251, "queue index"=0, "error in"=w255, "master data"="*Exit application", "queue in"=w256) -> ("error out"=w254:errorcluster, "queue out"=w253:T11)  [unwired: 5 in]
        n101 = event-data("Discard?"=TRUE) -> ()  [unwired: 1 in, 1 out]
      }
      event Value Change {
        w264 = u16 1 items=["HPRI"=1, "LPRI"=0] ("priority")
        n102 = event-data() -> ()  [unwired: 1 in, 6 out]
        n103 = call "Enqueue Element Array.vi"("priority"=w264, "queue index"=0, "error in"=w261, "master data"="Vision Paramter Save", "queue in"=w262) -> ("error out"=w259:errorcluster, "queue out"=w260:T11)  [unwired: 5 in]
      }
      event "取消按钮": Value Change {
        w271 = u16 1 items=["HPRI"=1, "LPRI"=0] ("priority")
        n104 = event-data() -> ()  [unwired: 1 in, 6 out]
        n105 = call "Enqueue Element Array.vi"("priority"=w271, "queue index"=0, "error in"=w268, "master data"="确认按钮", "queue in"=w269) -> ("error out"=w266:errorcluster, "queue out"=w267:T11)  [unwired: 5 in]
      }
      event "保存按钮": Value Change {
        w278 = u16 1 items=["HPRI"=1, "LPRI"=0] ("priority")
        n106 = event-data() -> ()  [unwired: 1 in, 6 out]
        n107 = call "Enqueue Element Array.vi"("priority"=w278, "queue index"=0, "error in"=w275, "master data"="程序参数保存", "queue in"=w276) -> ("error out"=w273:errorcluster, "queue out"=w274:T11)  [unwired: 5 in]
      }
      event "测试按钮": Value Change {
        w286 = u16 1 items=["HPRI"=1, "LPRI"=0] ("priority")
        n108 = event-data() -> ()  [unwired: 1 in, 6 out]
        n109 = property on="Main" class="TabCtl (严格)"("Value"=enum32{"主参数", "计算圆心参数 ", "边界检查器设定", "测试效果"}."测试效果" ("Main")) -> ()  [unwired: 2 in, 2 out]
        n110 = call "Enqueue Element Array.vi"("priority"=w286, "queue index"=0, "error in"=w283, "master data"="测试按钮", "queue in"=w284) -> ("error out"=w281:errorcluster, "queue out"=w282:T11)  [unwired: 5 in]
      }
      event "刷新": Value Change {
        n111 = event-data() -> ()  [unwired: 1 in, 6 out]
        n112 = disable-structure shown="禁用" {
          disable-tunnel: w292 -> [w296 _]
          disable-tunnel: w291 -> [w295 _]
          disable-tunnel: [w294 _] -> w290
          disable-tunnel: [w293 _] -> w289
          frame Disabled {
            w298 = u16 1 items=["HPRI"=1, "LPRI"=0] ("priority")
            # "刷新"
            n113 = call "Enqueue Element Array.vi"("priority"=w298, "queue index"=0, "error in"=w295, "master data"="刷新", "queue in"=w296) -> ("error out"=w293:errorcluster, "queue out"=w294:T11)  [unwired: 5 in]
          }
          frame Enabled {
          }
        }
        n114 = property on="Main" class="TabCtl (严格)"("Value"=enum32{"主参数", "计算圆心参数 ", "边界检查器设定", "测试效果"}."计算圆心参数 " ("Main")) -> ()  [unwired: 2 in, 2 out]
      }
    }
    n115 = call "GetSystemTime.vi"() -> ("date/time string"=→"system time":string)  [unwired: 7 in]
  }
  n116 = call "Release Queue Array.vi"("error in"=w4, "queue in"=w2) -> ("error out"=w3:errorcluster)  [unwired: 2 in, 3 out]
  n117 = call "Release Queue Array.vi"("error in"=w7, "queue in"=w2) -> ("error out"=w10:errorcluster)  [unwired: 2 in, 3 out]
  n118 = call "MergeErrors.vi"("error in 3 (no error)"=w3, "error in 4 (no error)"=w10) -> ("error out"=w9:errorcluster)  [unwired: 6 in]
  n119 = call "ExitAppMode.vi"("error in (no error)"=w9) -> ("error out"=w8:errorcluster)  [unwired: 10 in]
  n120 = call <vilib>:"Clear Errors.vi"("error in (no error)"=w8) -> ()  [unwired: 5 in, 2 out]
